vi "Wait for Valid Resource.vi"(8 "error in (no error)":errorcluster, 10 "timeout in ms (-1)":i32=-1, 11 "Generic Controller in":refnum<class "Generic Plugin.lvclass">) -> (0 "error out":errorcluster, 2 "Timeout?":bool, 3 "Generic Controller out":refnum<class "Generic Plugin.lvclass">)   [LabVIEW 2020, in "Generic Plugin.lvclass"]
uses:
  Generic Plugin.lvclass
  Generic Plugin.lvclass/Generic Plugin.ctl
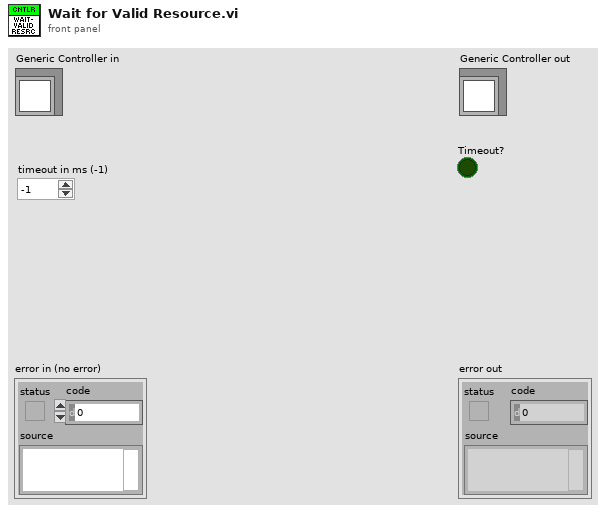
[diagram p1: front panel]
types:
  T1 = typedef "Dynamic Reentrant.lvlib/Message.ctl" = cluster{"Source":string, "Destination":string, "Time Stamp":timestamp, "Command":string, "Data":variant}
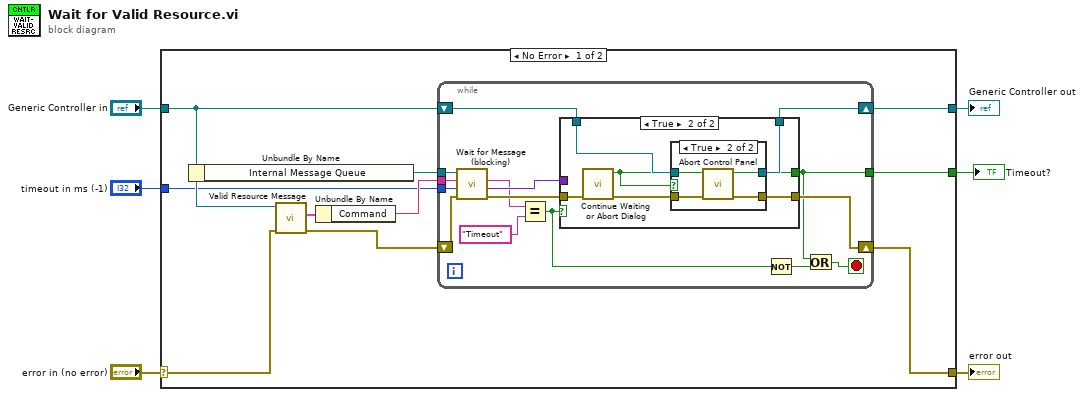
[diagram p0: block diagram]
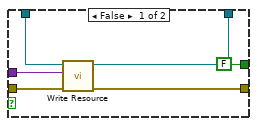
[diagram p2: hidden frame]
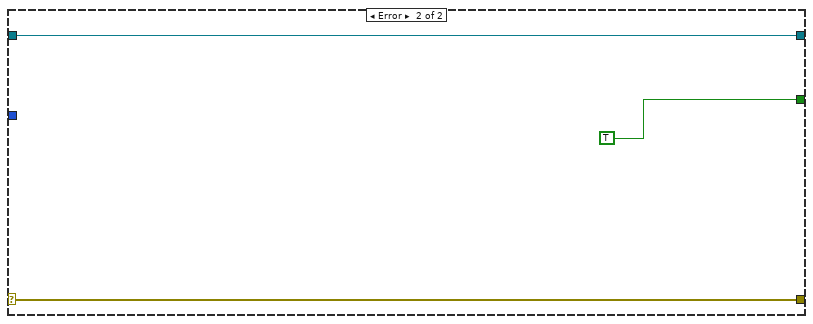
[diagram p4: hidden frame]
diagram:
  n1 = case shown="No Error" "error in (no error)" {
    selector: "error in (no error)" -> [w11 w52]
    tunnel: [w13 w52] -> w5
    tunnel: [w9 w51] -> w3
    tunnel: "Generic Controller in" -> [w10 w51]
    tunnel: [w8 TRUE] -> w2
    tunnel: "timeout in ms (-1)" -> [w7 _]
    frame No Error {
      n2 = Unbundle By Name(w10) -> ("Internal Message Queue"=w16:refnum<queue>)
      n3 = call-dynamic "Valid Resource Message.vi"("error in (no error)"=w11, "Generic Controller in"=w10) -> ("error out"=w12:errorcluster, "Valid Resource Message"=w15:T1)  [unwired: 7 in, 1 out]
      n4 = Unbundle By Name(w15) -> ("Command"=w14:string)
      n5 = while {
        tunnel: w16 -> [w31]
        tunnel: w14 -> [w30]
        tunnel: [w17] -> w8
        tunnel: w7 -> [w21]
        shift-right: [w27] -> w13
        shift-left: w12 -> [w26]
        shift-right: [w24] -> w9
        shift-left: w10 -> [w25]
        stop <- w20 stop-if-true
        n6 = call "Wait for Message (blocking).vi"("error in (no error)"=w26, "timeout in ms (-1)"=w21, "Command"=w30, "Listening queue in"=w31) -> ("error out"=w28:errorcluster, "Message Data"=w29:variant, "Message"=w22:string)  [unwired: 4 in, 1 out]
        n7 = Equal?(x=w22, y="Timeout") -> (x = y?=w19:bool)
        n8 = case shown="True" w19 {
          tunnel: w29 -> [w37 _]
          tunnel: w28 -> [w36 w43]
          tunnel: [w35 w41] -> w27
          tunnel: w25 -> [w34 w40]
          tunnel: [w33 w39] -> w24
          tunnel: [FALSE ("Abort?") w38] -> w17
          frame False {
            n9 = call-dynamic "Write Resource.vi"("error in (no error)"=w36, "Resource"=w37, "Generic Controller in"=w34) -> ("error out"=w35:errorcluster, "Generic Controller out"=w33:refnum<class "Generic Plugin.lvclass">)  [unwired: 7 in]
          }
          frame True {
            n10 = call "Continue Waiting or Abort Dialog.vi"("error in (no error)"=w43) -> ("error out"=w42:errorcluster, "Abort?"=w38:bool)  [unwired: 9 in]
            n11 = case shown="True" w38 {
              tunnel: w42 -> [w44 w49]
              tunnel: [w44 w48] -> w41
              tunnel: w40 -> [w45 w47]
              tunnel: [w45 w46] -> w39
              frame False {
              }
              frame True {
                n12 = call "Abort Control Panel.vi"("error in (no error)"=w49, "Generic Controller in"=w47) -> ("error out"=w48:errorcluster, "Generic Controller out"=w46:refnum<class "Generic Plugin.lvclass">)  [unwired: 8 in]
              }
            }
          }
        }
        n13 = Not(x=w19) -> (.not. x?=w18:bool)
        n14 = Or(x=w17, y=w18) -> (x .or. y?=w20:bool)
      }
    }
    frame Error {
    }
  }
  "error out" <- w5
  "Generic Controller out" <- w3
  "Timeout?" <- w2
